vi "Auto Command Executor.vi"() -> (3 "Done Executing Command":bool)   [LabVIEW 2017]
uses:
  Cube Manipulation Controls.ctl
  Cube Manipulation Manual Controls.ctl
  Robot Global Data.vi
  <vilib>/Rock Robotics/WPI/Solenoid/Deprecated/WPI_SolenoidSetBool.vi
  <vilib>/Rock Robotics/WPI/Solenoid/Deprecated/WPI_SolenoidGetBool.vi
panel:
  in  "Carrage Contiunous voltage":dbl=-1.0
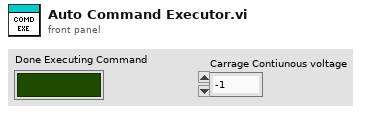
[diagram p1: front panel]
types:
  T1 = typedef "Cube Manipulation Manual Controls.ctl" = cluster{"Extend Long Solinoid":bool, "Retract Long Solinoid":bool, "Extend Short Solinoid":bool, "Retract Short Solinoid":bool, "Override Lift Control":bool, "Override Intake Control":bool, "Clear Intake Area":bool}
  T2 = typedef "Cube Manipulation Controls.ctl" = cluster{"Intake Sequence":bool, "Switch Position":bool, "Scale Position Low":bool, "Scale Position Mid":bool, "Scale Position High":bool, "Re-adjust Grip":bool, "Manual Mode":bool, "Manual Toggle Long":bool, "Manual Toggle Short":bool, "Eject Cube":bool, "Manual Lift Control":bool, "Exchange Sequence":bool, "Open Intk Short 4 Intk":bool, "Slow Eject":bool}
  T3 = typedef "Cube Manipulation Outputs.ctl" = cluster{"Control Mode":T4, "Carrage Output":dbl, "Intake Output":dbl, "Intake Short":bool, "Intake Long":bool, "Lift Output":dbl, "Lift Output L":dbl, "Lift Output R":dbl}
  T4 = typedef "CTRE_Phoenix_MotorControl_ControlMode.ctl" = u16
  T5 = typedef "WPI_MotorControlDeviceRef.ctl" = cluster{"DeviceStatus":errorcluster, "Type":T6, "PWM":cluster{"PWM Channel":T7, "DeadBand":T8}, "CAN":cluster{"Device Number":u8, "SetOutput VI Ref":variant, "GetOutput VI Ref":variant, "Enable VI Ref":variant, "Disable VI Ref":variant, "Data":variant}, "Invert":bool, "DIO PWM":cluster{"PWM \"Enable\" Channel":T7, "DIOChannel":T9, "PWM Rate":dbl}}
  T6 = typedef "WPI_MotorControlType.ctl" = enum16{"PWM", "CAN", "DIO PWM"}
  T7 = typedef "FPGA_DIOPWMChannel.ctl" = enum8{"PWM 0", "PWM 1", "PWM 2", "PWM 3", "PWM 4", "PWM 5", "PWM 6", "PWM 7", "PWM 8", "PWM 9", "PWM MXP 0", "PWM MXP 1", "PWM MXP 2", "PWM MXP 3", "PWM MXP 4", "PWM MXP 5", "PWM MXP 6", "PWM MXP 7", "PWM MXP 8", "PWM MXP 9", "Invalid"}
  T8 = typedef "WPI_PWMDeadband.ctl" = cluster{"Name":string, "maxPositivePwm":i32, "minPositivePwm":i32, "centerPwm":i32, "maxNegativePwm":i32, "minNegativePwm":i32, "angularRange":u16}
  T9 = typedef "FPGA_DIOChannel.ctl" = enum8{"DIO 0", "DIO 1", "DIO 2", "DIO 3", "DIO 4", "DIO 5", "DIO 6", "DIO 7", "DIO 8", "DIO 9", "DIO MXP 0", "DIO MXP 1", "DIO MXP 2", "DIO MXP 3", "DIO MXP 4", "DIO MXP 5", "DIO MXP 6", "DIO MXP 7", "DIO MXP 8", "DIO MXP 9", "DIO MXP 10", "DIO MXP 11", "DIO MXP 12", "DIO MXP 13", "DIO MXP 14", "DIO MXP 15", "SPI Port CS1", "SPI Port CS2", "SPI Port CS3", "SPI Port MISO", "SPI Port MOSI", "Invalid"}
  T10 = typedef "WPI_SolenoidDevRef.ctl" = cluster{"DevStatus":errorcluster, "Pneumatics Control Module":u8, "Forward Solenoid Channel":T11, "Reverse Solenoid Channel":T11}
  T11 = typedef "WPI_SolenoidChannel.ctl" = enum8{"Solenoid 0", "Solenoid 1", "Solenoid 2", "Solenoid 3", "Solenoid 4", "Solenoid 5", "Solenoid 6", "Solenoid 7", "Invalid"}
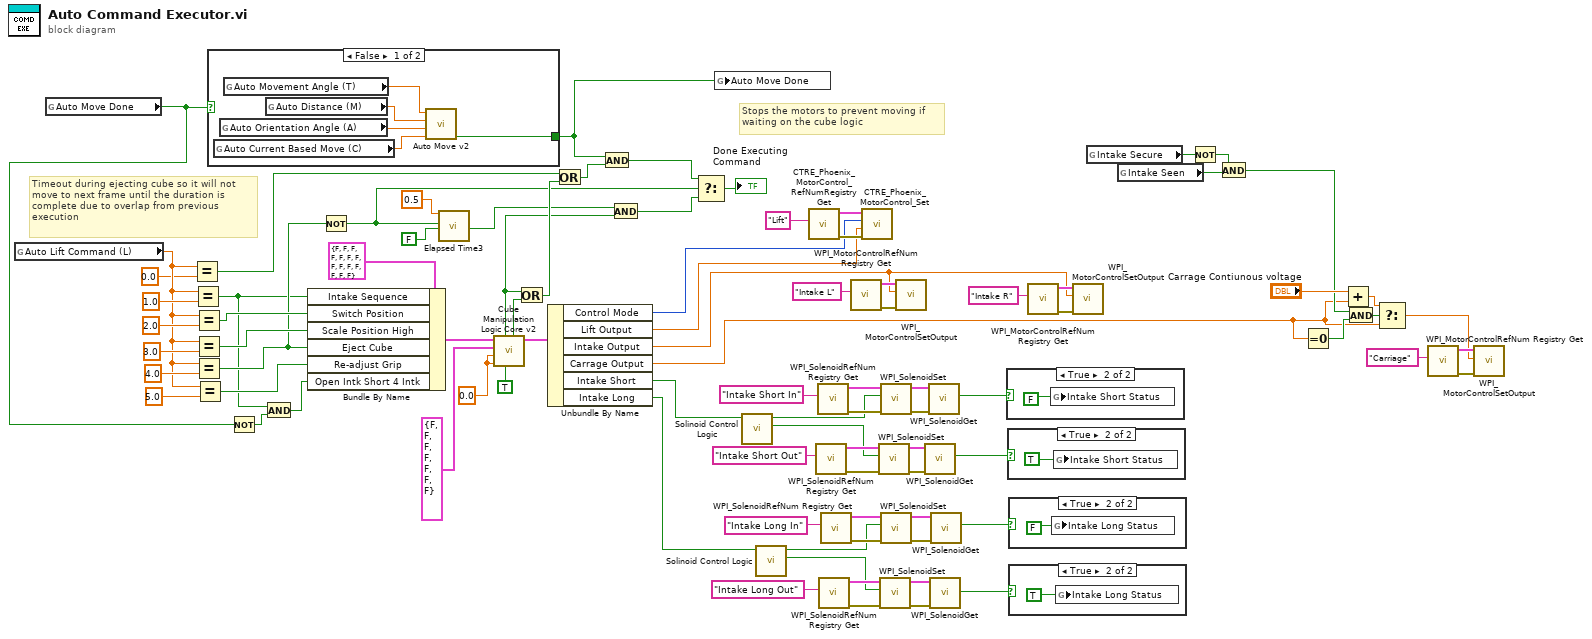
[diagram p0: block diagram]
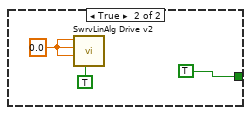
[diagram p2: hidden frame]
diagram:
  w25 = 0.0 ("Manual Lift Control")
  # "Stops the motors to prevent moving if\nwaiting on the cube logic"
  # "Timeout during ejecting cube so it will not\nmove to next frame until the duration is\ncomplete due to overlap from previous\nexecution"
  n1 = global read "Robot Global Data.vi" "Auto Lift Command (L)"() -> (w36:dbl)
  n2 = global read "Robot Global Data.vi" "Auto Move Done"() -> (w1:bool)
  n3 = Equal?(x=w36, y=0.0) -> (x = y?=w32:bool)
  n4 = Equal?(x=w36, y=1.0) -> (x = y?=w3:bool)
  n5 = Equal?(x=w36, y=2.0) -> (x = y?=w46:bool)
  n6 = Equal?(x=w36, y=3.0) -> (x = y?=w45:bool)
  n7 = Equal?(x=w36, y=4.0) -> (x = y?=w20:bool)
  n8 = Equal?(x=w36, y=5.0) -> (x = y?=w44:bool)
  n9 = case shown="False" w1 {
    tunnel: [w94 TRUE ("Done")] -> w30
    frame False {
      n10 = global read "Robot Global Data.vi" "Auto Current Based Move (C)"() -> (w90:dbl)
      n11 = global read "Robot Global Data.vi" "Auto Orientation Angle (A)"() -> (w91:dbl)
      n12 = global read "Robot Global Data.vi" "Auto Movement Angle (T)"() -> (w93:dbl)
      n13 = global read "Robot Global Data.vi" "Auto Distance (M)"() -> (w92:dbl)
      n14 = call "Auto Move v2.vi"("Current Based Move"=w90, "Orientation Angle"=w91, "Move Distance"=w92, "Movement Angle"=w93) -> ("Done Moving"=w94:bool)  [unwired: 7 in]
    }
    frame True {
      w95 = 0.0 ("X")
      n15 = call "SwrvLinAlg Drive v2.vi"("Auto Controls"=TRUE, "Z"=w95, "Y"=w95, "X"=w95) -> ()  [unwired: 8 in]
    }
  }
  n16 = Not(x=w1) -> (.not. x?=w2:bool)
  n17 = And(x=w3, y=w2) -> (x .and. y?=w4:bool)
  n18 = Bundle By Name(cluster=T2 {"Intake Sequence"=FALSE, "Switch Position"=FALSE, "Scale Position Low"=FALSE, "Scale Position Mid"=FALSE, "Scale Position High"=FALSE, "Re-adjust Grip"=FALSE, "Manual Mode"=FALSE, "Manual Toggle Long"=FALSE, "Manual Toggle Short"=FALSE, "Eject Cube"=FALSE, "Manual Lift Control"=FALSE, "Exchange Sequence"=FALSE, "Open Intk Short 4 Intk"=FALSE, "Slow Eject"=FALSE} ("Cube Manipulation Controls"), "Intake Sequence"=w3, "Switch Position"=w46, "Scale Position High"=w45, "Eject Cube"=w20, "Re-adjust Grip"=w44, "Open Intk Short 4 Intk"=w4) -> (w88:T2)
  n19 = Not(x=w20) -> (.not. x?=w8:bool)
  n20 = call "Elapsed Time3"("Time Target (s)"=0.5, "Reset"=w8, "Auto Reset"=FALSE) -> ("Time has Elapsed"=w19:bool)  [unwired: 9 in, 7 out]
  n21 = call "Cube Manipulation Logic Core v2.vi"("Auto Control"=TRUE, "Manual Intake Control"=w25, "Manual Lift Control"=w25, "Cube Manipulation Manual Controls"=T1 {"Extend Long Solinoid"=FALSE, "Retract Long Solinoid"=FALSE, "Extend Short Solinoid"=FALSE, "Retract Short Solinoid"=FALSE, "Override Lift Control"=FALSE, "Override Intake Control"=FALSE, "Clear Intake Area"=FALSE}, "Cube Manipulation Button Controls"=w88) -> ("output cluster"=w87:T3, "Sequence Done"=w38:bool, "Position Reached"=w23:bool)  [unwired: 4 in]
  n22 = Or(x=w23, y=w38) -> (x .or. y?=w33:bool)
  n23 = Unbundle By Name(w87) -> ("Control Mode"=w47:T4, "Lift Output"=w48:dbl, "Intake Output"=w26:dbl, "Carrage Output"=w10:dbl, "Intake Short"=w58:bool, "Intake Long"=w57:bool)
  n24 = Or(x=w32, y=w33) -> (x .or. y?=w34:bool)
  n25 = And(x=w30, y=w34) -> (x .and. y?=w5:bool)
  n26 = And(x=w19, y=w23) -> (x .and. y?=w7:bool)
  n27 = Select(t=w5, s=w8, f=w7) -> (s? t:f=→"Done Executing Command":bool)
  n28 = global write "Robot Global Data.vi" "Auto Move Done"(w30) -> ()
  n29 = call "Solinoid Control Logic.vi"("Input"=w58) -> ("Out"=w59:bool, "In"=w60:bool)  [unwired: 9 in]
  n30 = call "Solinoid Control Logic.vi"("Input"=w57) -> ("Out"=w61:bool, "In"=w62:bool)  [unwired: 9 in]
  n31 = call "CTRE_Phoenix_MotorControl_RefNumRegistryGet.vi"("refnum name"="Lift") -> ("error out"=w49:errorcluster, "PhoenixMotorControlDevRef"=w50:T5)  [unwired: 9 in]
  n32 = call <vilib>:"WPI_SolenoidRefNum Registry Get.vi"("refnum name"="Intake Short Out") -> ("error out"=w76:errorcluster, "SolenoidDevRef"=w75:T10)  [unwired: 9 in]
  n33 = call <vilib>:"WPI_SolenoidRefNum Registry Get.vi"("refnum name"="Intake Short In") -> ("error out"=w78:errorcluster, "SolenoidDevRef"=w77:T10)  [unwired: 9 in]
  n34 = call <vilib>:"WPI_SolenoidRefNum Registry Get.vi"("refnum name"="Intake Long Out") -> ("error out"=w80:errorcluster, "SolenoidDevRef"=w79:T10)  [unwired: 9 in]
  n35 = call <vilib>:"WPI_SolenoidRefNum Registry Get.vi"("refnum name"="Intake Long In") -> ("error out"=w82:errorcluster, "SolenoidDevRef"=w81:T10)  [unwired: 9 in]
  n36 = call <vilib>:"WPI_MotorControlRefNum Registry Get.vi"("refnum name"="Intake L") -> ("error out"=w27:errorcluster, "MotorControlDevRef"=w28:T5)  [unwired: 9 in]
  n37 = call <vilib>:"CTRE_Phoenix_MotorControl_Set.vi"("error in (no error)"=w49, "Output"=w48, "Control Mode"=w47, "PhoenixMotorControlDevRef"=w50) -> ()  [unwired: 6 in, 2 out]
  n38 = call-poly <vilib>:"WPI_SolenoidSet.vi"("error in (no error)"=w76, "Value"=w59, "SolenoidDevRef"=w75) -> ("error out"=w68:errorcluster, "SolenoidDevRef"=w67:T10)  [unwired: 7 in]
  n39 = call-poly <vilib>:"WPI_SolenoidSet.vi"("error in (no error)"=w80, "Value"=w61, "SolenoidDevRef"=w79) -> ("error out"=w72:errorcluster, "SolenoidDevRef"=w71:T10)  [unwired: 7 in]
  n40 = call-poly <vilib>:"WPI_SolenoidSet.vi"("error in (no error)"=w78, "Value"=w60, "SolenoidDevRef"=w77) -> ("error out"=w70:errorcluster, "SolenoidDevRef"=w69:T10)  [unwired: 7 in]
  n41 = call-poly <vilib>:"WPI_SolenoidSet.vi"("error in (no error)"=w82, "Value"=w62, "SolenoidDevRef"=w81) -> ("error out"=w74:errorcluster, "SolenoidDevRef"=w73:T10)  [unwired: 7 in]
  n42 = call <vilib>:"WPI_MotorControlSetOutput.vi"("error in (no error)"=w27, "Output"=w26, "MotorControlDevRef"=w28) -> ()  [unwired: 6 in, 3 out]
  n43 = call-poly <vilib>:"WPI_SolenoidGet.vi"("error in (no error)"=w68, "SolenoidDevRef"=w67) -> ("Value"=w65:bool)  [unwired: 7 in, 2 out]
  n44 = call-poly <vilib>:"WPI_SolenoidGet.vi"("error in (no error)"=w70, "SolenoidDevRef"=w69) -> ("Value"=w64:bool)  [unwired: 7 in, 2 out]
  n45 = call-poly <vilib>:"WPI_SolenoidGet.vi"("error in (no error)"=w72, "SolenoidDevRef"=w71) -> ("Value"=w63:bool)  [unwired: 7 in, 2 out]
  n46 = call-poly <vilib>:"WPI_SolenoidGet.vi"("error in (no error)"=w74, "SolenoidDevRef"=w73) -> ("Value"=w66:bool)  [unwired: 7 in, 2 out]
  n47 = case shown="True" w64 {
    frame False {
    }
    frame True {
      n48 = global write "Robot Global Data.vi" "Intake Short Status"(FALSE ("Intake Short Status")) -> ()
    }
  }
  n49 = case shown="True" w65 {
    frame False {
    }
    frame True {
      n50 = global write "Robot Global Data.vi" "Intake Short Status"(TRUE ("Intake Short Status")) -> ()
    }
  }
  n51 = case shown="True" w66 {
    frame False {
    }
    frame True {
      n52 = global write "Robot Global Data.vi" "Intake Long Status"(FALSE ("Intake Long Status")) -> ()
    }
  }
  n53 = case shown="True" w63 {
    frame False {
    }
    frame True {
      n54 = global write "Robot Global Data.vi" "Intake Long Status"(TRUE ("Intake Long Status")) -> ()
    }
  }
  n55 = call <vilib>:"WPI_MotorControlRefNum Registry Get.vi"("refnum name"="Intake R") -> ("error out"=w56:errorcluster, "MotorControlDevRef"=w55:T5)  [unwired: 9 in]
  n56 = call <vilib>:"WPI_MotorControlSetOutput.vi"("error in (no error)"=w56, "Output"=w26, "MotorControlDevRef"=w55) -> ()  [unwired: 6 in, 3 out]
  n57 = global read "Robot Global Data.vi" "Intake Secure"() -> (w14:bool)
  n58 = global read "Robot Global Data.vi" "Intake Seen"() -> (w16:bool)
  n59 = Not(x=w14) -> (.not. x?=w15:bool)
  n60 = And(x=w15, y=w16) -> (x .and. y?=w12:bool)
  n61 = Equal To 0?(x=w10) -> (x = 0?=w11:bool)
  n62 = Add(x="Carrage Contiunous voltage", y=w10) -> (x+y=w18:dbl)
  n63 = And(x=w12, y=w11) -> (x .and. y?=w13:bool)
  n64 = Select(t=w18, s=w13, f=w10) -> (s? t:f=w9:dbl)
  n65 = call <vilib>:"WPI_MotorControlRefNum Registry Get.vi"("refnum name"="Carriage") -> ("error out"=w52:errorcluster, "MotorControlDevRef"=w37:T5)  [unwired: 9 in]
  n66 = call <vilib>:"WPI_MotorControlSetOutput.vi"("error in (no error)"=w52, "Output"=w9, "MotorControlDevRef"=w37) -> ()  [unwired: 6 in, 3 out]
